vi "判断追溯码.vi"(9 "当前设备编号":string, 10 "前序设备编号":string, 11 "追溯码":string) -> (3 "追溯码有效":bool)   [LabVIEW 2018]
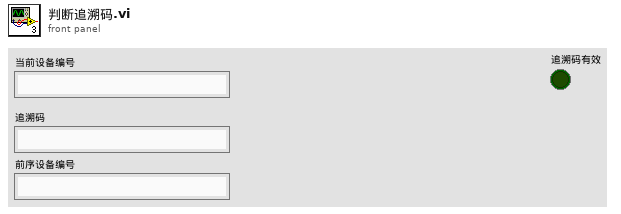
[diagram p1: front panel]
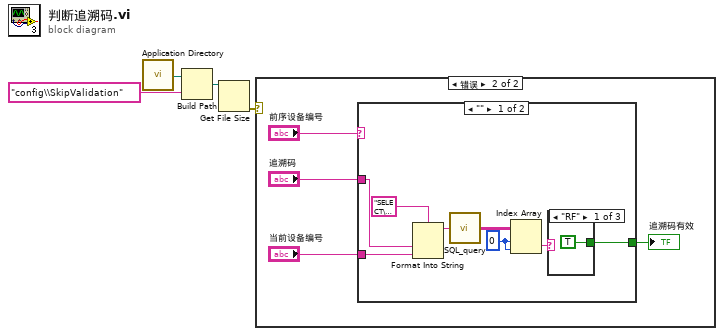
[diagram p0: block diagram]
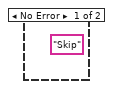
[diagram p2: hidden frame]
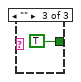
[diagram p4: hidden frame]
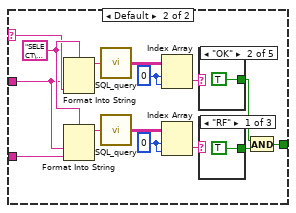
[diagram p5: hidden frame]
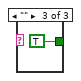
[diagram p7: hidden frame]
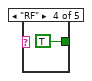
[diagram p10: hidden frame]
diagram:
  n1 = call <vilib>:"Application Directory.vi"() -> ("Application Directory"=w4:path)
  n2 = Build Path(base path=w4, name or relative path="config\\SkipValidation" ("名称或相对路径")) -> (appended path=w2:path)
  n3 = Get File Size(file=w2) -> (0:w1:errorcluster)  [unwired: 1 in, 2 out]
  n4 = case shown="错误" w1 {
    frame No Error {
      (unwired) "Skip"
    }
    frame Error {
      n5 = case shown="\"\"" "前序设备编号" {
        selector: "前序设备编号" -> [_ w22]
        tunnel: "当前设备编号" -> [w10 w21]
        tunnel: "追溯码" -> [w11 w20]
        tunnel: [w9 w19] -> w5
        frame "" {
          w14 = 0 ("索引 (行)")
          n6 = Format Into String(format string="SELECT\n\tdbo.[产品质量1].[加工状态]\nFROM\n\tdbo.[产品质量1]\nWHERE\n\tdbo.[产品质量1].[工位追溯码] = '%s'\nAND dbo.[产品质量1].[设备编号] = '%s'\n", w11, w10) -> (resulting string=w15:string)  [unwired: 2 in, 1 out]
          n7 = call "SQL_query.vi"("SQL query"=w15) -> ("data"=w13:string[][])  [unwired: 2 in, 2 out]
          n8 = Index Array(array=w13, index (row)=w14, index (col)=w14) -> (element=w12:string)
          n9 = case shown="\"RF\"" w12 {
            tunnel: [TRUE _ TRUE] -> w9
            frame "RF" {
            }
            frame Default {
            }
            frame "" {
            }
          }
        }
        frame Default {
          w28 = 0 ("索引 (行)")
          w31 = 0 ("索引 (行)")
          w30 = "SELECT\n\tdbo.[产品质量1].[加工状态]\nFROM\n\tdbo.[产品质量1]\nWHERE\n\tdbo.[产品质量1].[工位追溯码] = '%s'\nAND dbo.[产品质量1].[设备编号] = '%s'\n"
          n10 = Format Into String(format string=w30, w20, w22) -> (resulting string=w33:string)  [unwired: 2 in, 1 out]
          n11 = Format Into String(format string=w30, w20, w21) -> (resulting string=w29:string)  [unwired: 2 in, 1 out]
          n12 = call "SQL_query.vi"("SQL query"=w33) -> ("data"=w32:string[][])  [unwired: 2 in, 2 out]
          n13 = call "SQL_query.vi"("SQL query"=w29) -> ("data"=w27:string[][])  [unwired: 2 in, 2 out]
          n14 = Index Array(array=w32, index (row)=w31, index (col)=w31) -> (element=w23:string)
          n15 = Index Array(array=w27, index (row)=w28, index (col)=w28) -> (element=w24:string)
          n16 = case shown="\"OK\"" w23 {
            tunnel: [_ TRUE _ TRUE _] -> w26
            frame Default {
            }
            frame "OK" {
            }
            frame "NG" {
            }
            frame "RF" {
            }
            frame "WG" {
            }
          }
          n17 = case shown="\"RF\"" w24 {
            tunnel: [TRUE _ TRUE] -> w25
            frame "RF" {
            }
            frame Default {
            }
            frame "" {
            }
          }
          n18 = And(x=w26, y=w25) -> (x .and. y?=w19:bool)
        }
      }
      "追溯码有效" <- w5
    }
  }
